vi "FPGA VI.vi"() -> ()   [LabVIEW 2015]
uses:
  Types/Injector.Timing.ctl
  Types/Injection.Core.Settings.ctl
  Types/Injection.Global.Settings.ctl
  <vilib>/rvi/eio/common/nirviEmuClasses.ctl
  <vilib>/Platform/TimedLoop/XDataNode/timing_clust.ctl
  <vilib>/Platform/TimedLoop/XDataNode/nitl_modes.ctl
  <vilib>/Platform/TimedLoop/XDataNode/wakeup.ctl
  Types/Injection.Core.Internal.Settings.ctl
  <vilib>/rvi/eio/common/nirviEmuTemplateMethod_errors.vi
  <vilib>/rvi/Emulation/niFpgaGetClockAttributes.vi
  <vilib>/rvi/Emulation/niFpgaSctlEmulationGetInTimedLoop.vi
  <vilib>/rvi/Emulation/niFpgaEmulationReportErrorSimple.vi
  <vilib>/rvi/Emulation/niFpgaCriticalErrorInLSC.vi
  <vilib>/rvi/DataTransferAndStorage/Container/Common/niFpgaContainerExecOnDevCompGetState.vi
  <vilib>/rvi/Emulation/niFpgaEmulationIsFPGAContextNoSignature.vi
  <vilib>/rvi/errors/niFpgaSetErrorForExecOnDevCompSimple.vi
  <vilib>/rvi/eio/common/nirviEmuReportErrorAndStop.vi
  <vilib>/rvi/DataTransferAndStorage/Container/Common/niFpgaContainerGetUniqueNameForEmu.vi
  <vilib>/rvi/FIFO/Fifo_Resource/nirvififoEmulationSetSize.vi
  <vilib>/rvi/FIFO/Fifo_Resource/nirviFifoEmulationQueueMgr.vi
  <instcachedir>/0/nirviFifoEmulationQueueMgr_E5CAEC123FF24DC58D834DCA3CDAA9B5.lvgen/nirviFifoEmulationQueueMgr_E5CAEC123FF24DC58D834DCA3CDAA9B5_010.vi
  <vilib>/rvi/FIFO/Fifo_Resource/nirvififoEmulationDetermineInputValidOut.vi
  <vilib>/rvi/FIFO/Fifo_Resource/nirvififoEmulationCreateLock.vi
  <vilib>/rvi/Emulation/niFpgaProcessEmulError.vi
  <vilib>/rvi/FIFO/Fifo_Resource/nirvififoEmulationObtainLock.vi
  <vilib>/rvi/FIFO/Fifo_Resource/nirvififoEmulationReleaseLock.vi
  <vilib>/rvi/occurrence/nirviWaitOnOccurrenceBase.vi
  <vilib>/rvi/errors/nirviReportUnexpectedCaseInternalError.vi
  <vilib>/rvi/errors/nirviReportUnexpectedCaseInternalError (U32).vi
  <vilib>/Utility/error.llb/Clear Errors.vi
  <vilib>/rvi/interface/RandomDataEmulation/niFpgaRandomDataHandleErrors.vi
  <instcachedir>/0/nirviFifoEmulationQueueMgr_E5CAEC123FF24DC58D834DCA3CDAA9B5.lvgen/nirviFifoEmulationQueueMgr_E5CAEC123FF24DC58D834DCA3CDAA9B5_008.vi
  <vilib>/eio/EIOGrowableMethodNode/genericMethod/EIOGrowableMethodNode.xnode
  <vilib>/rvi/eio/nirviEIOMethodImplementation/nirviEIOMethodImplementation.xnode
  <vilib>/rvi/eio/nirviErrorMerge/nirviErrorMerge.xnode
  <vilib>/eio/EIONode/EIONode.xnode
  <vilib>/Platform/TimedLoop/XDataNode/XDataNode.xnode
  <vilib>/rvi/DataTransferAndStorage/Container/XNode/niFpgaContainer.xnode
  <vilib>/rvi/FIFO/Fifo_Resource/niFpgaFifoEmulationRefIn.vi
  <vilib>/rvi/interface/RandomDataEmulation/nirviRandomDataFpgaReadWriteTemplate.vi
  <vilib>/Platform/TimedLoop/XDataNode/XDNodeRunTimeDep.lvlib
  <vilib>/rvi/eio/common/nirviEmuTemplateMethod_noerrors.vi
panel:
  out "Module Error":bool
  out "Sample Clock Ticks":u32
  out "Intermediate FIFO Write Timeout":bool
  in  "Settings.Global":T1={"Enable?"=FALSE, "Initial Voltage Threshold"=12.0, "Event Dwell Limit"=2000, "Voltage Gain"=1.0, "Current Gain"=1.0}
  in  "Settings.Index0.Injector0":T2
  in  "Settings.Index1.Injector1":T2
  in  "Settings.Index2.Injector2":T2
  in  "Settings.Index3.Injector3":T2
  in  "Settings.Index4.Injector4":T2
  in  "Settings.Index5.Injector5":T2
  in  "Settings.Timing":T3={"Injector Sample Period (Ticks)"=200}
  out "Acqusition Loop Ticks":u32
  in  "Settings.DMA":cluster{"# of Injectors":u8}={"# of Injectors"=6}
  out "Host DMA Out?":bool
  out "Intermediate Time Out?":bool
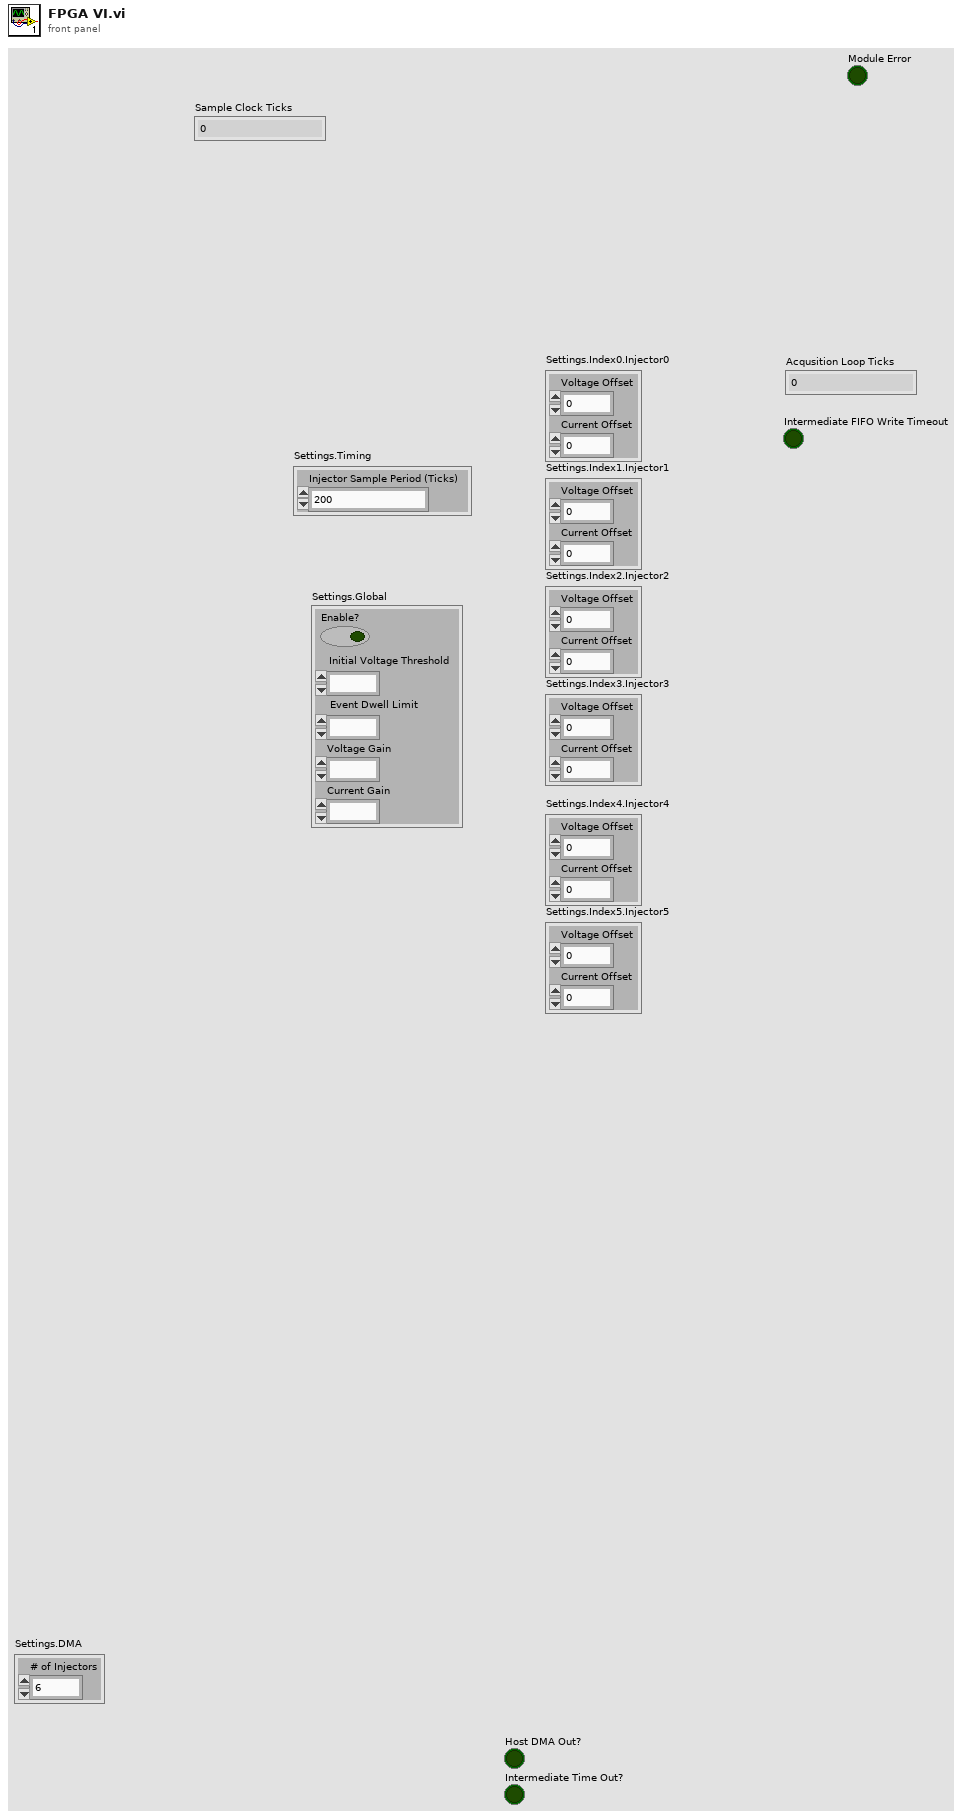
[diagram p1: front panel]
types:
  T1 = typedef "Injection.Global.Settings.ctl" = cluster{"Enable?":bool, "Initial Voltage Threshold":fxp<+/-,32,8>, "Event Dwell Limit":u16, "Voltage Gain":fxp<+/-,32,8>, "Current Gain":fxp<+/-,32,8>}
  T2 = typedef "Injection.Core.Settings.ctl" = cluster{"Voltage Offset":fxp<+/-,32,8>, "Current Offset":fxp<+/-,32,8>}
  T3 = typedef "Injector.Timing.ctl" = cluster{"Injector Sample Period (Ticks)":u32}
  T4 = typedef "nirviEmuClasses.ctl" = enum16{"IO Read", "IO Write", "Method", "Property Read", "Property Write"}
  T5 = cluster{"Data.Samples":u32, "Injection.Period":u32, "Injector.Index":u8, "Iteration":u32}
  T6 = enum8{"Wait on Transfer", "Transfer Injector Index", "Transfer # of Samples", "Transfer Injection Period", "Transfer Data Samples"}
  T7 = typedef "XDNodeRunTimeDep.lvlib/timing_clust.ctl" = cluster{"Expected End [f-1]":u64, "Actual End [f-1]":u64, "Finished Late? [f-1]":bool, "Expected End [i-1]":u64, "Actual End [i-1]":u64, "Finished Late? [i-1]":bool, "Expected Start [i]":u64, "Actual Start [i]":u64, "Expected Start [f]":u64, "Actual Start [f]":u64, "Source Name":string, "Structure Name":string, "Period":i64, "Deadline":i64, "Offset":i64, "Start":i64, "Priority":i32, "Timeout":i32, "Mode":T8, "Wakeup Reason":T9, "Error":errorcluster, "Source Type":string, "Secondary Source Type":string, "Global End Time":u64, "Global Start Time":u64, "Frame Duration":u64, "Iteration Duration":u64, "Assigned CPU":i32, "I/O Scan Engine Mode":u32}
  T8 = typedef "XDNodeRunTimeDep.lvlib/nitl_modes.ctl" = enum32{"No Change", "Process missed periods, maintain original phase", "Discard missed periods, maintain original phase", "Process missed periods, ignore original phase", "Discard missed periods, ignore original phase"}
  T9 = typedef "XDNodeRunTimeDep.lvlib/wakeup.ctl" = enum32{"Normal", "Aborted", "Asynchronous wakeup", "Timing source error", "Timed loop error", "Timeout"}
  T10 = typedef "Injection.Core.Internal.Settings.ctl" = cluster{"Data FIFO":refnum<k21>, "Trigger FIFO":refnum<k21>}
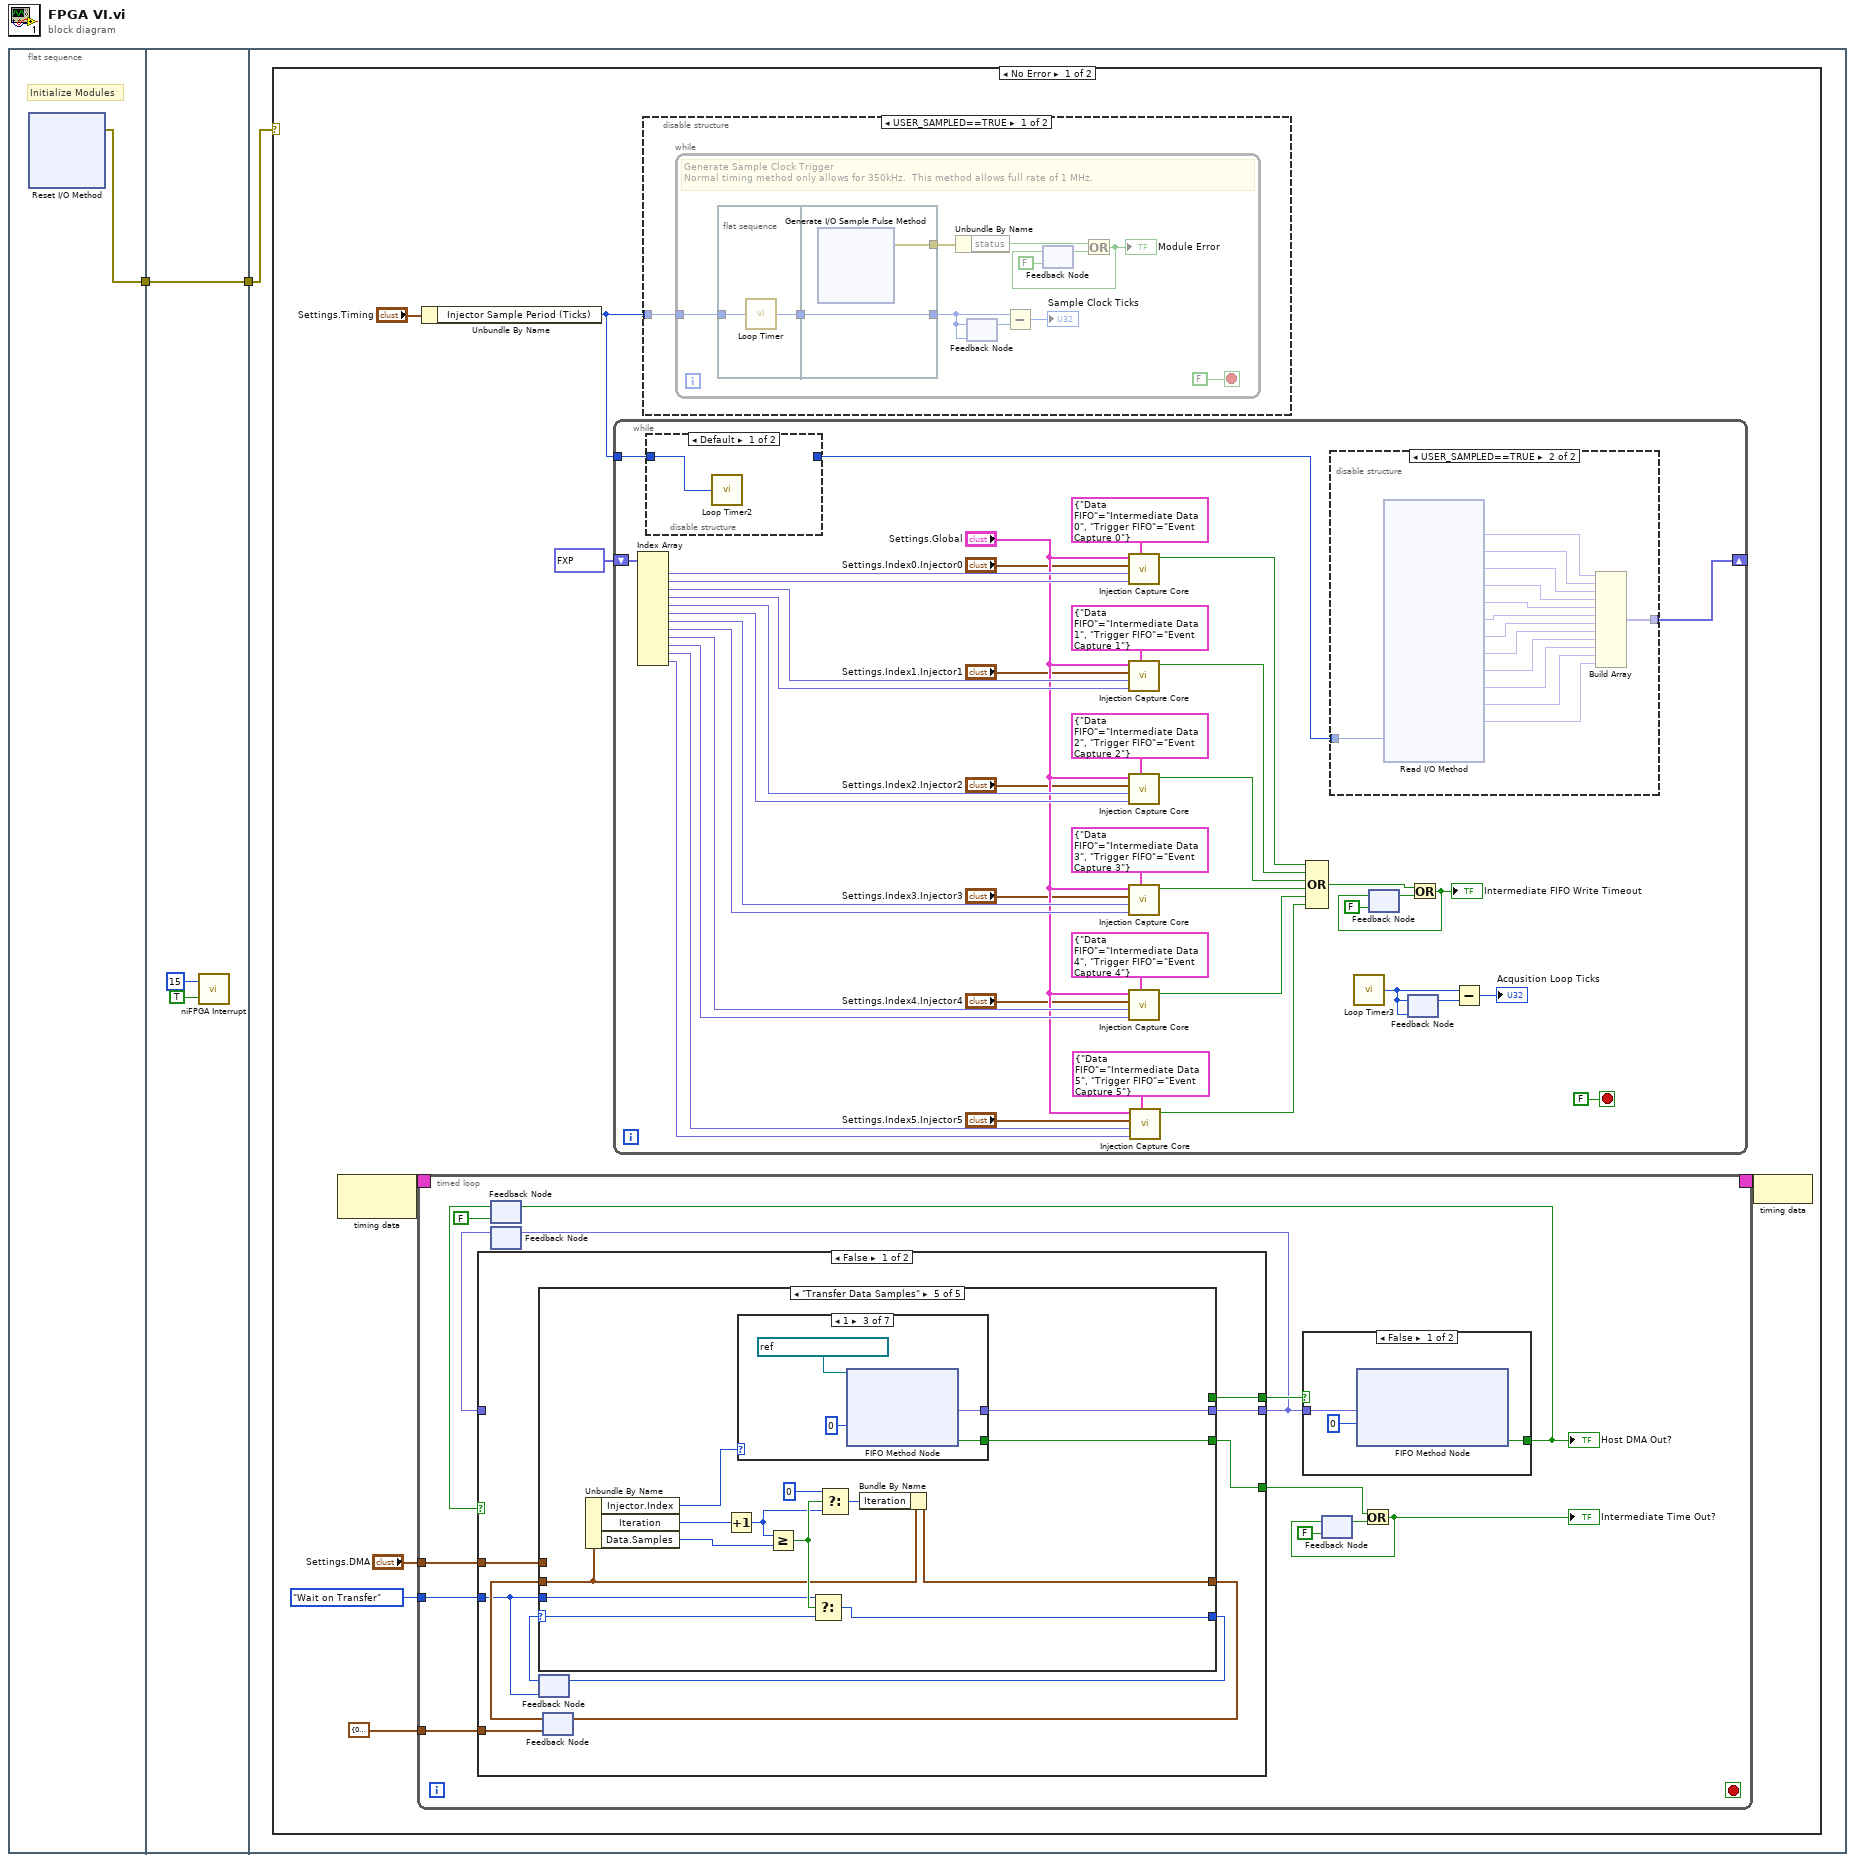
[diagram p0: block diagram]
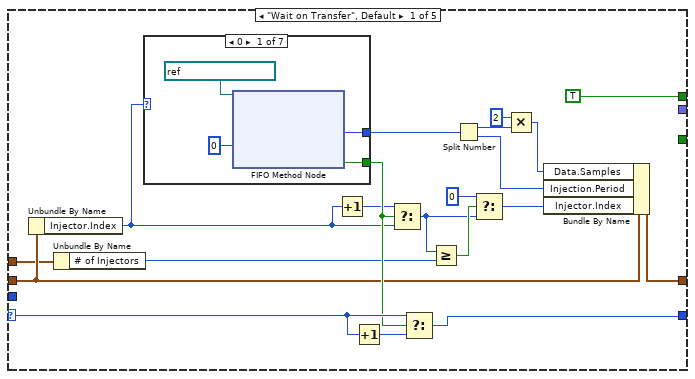
[diagram p2: hidden frame]
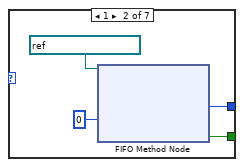
[diagram p3: hidden frame]
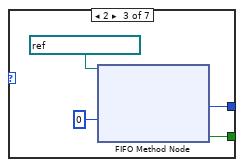
[diagram p4: hidden frame]
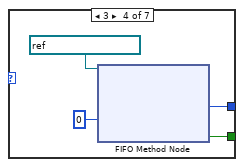
[diagram p5: hidden frame]
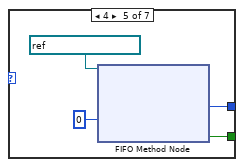
[diagram p6: hidden frame]
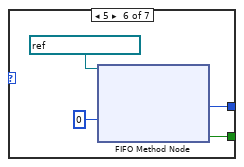
[diagram p7: hidden frame]
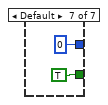
[diagram p8: hidden frame]
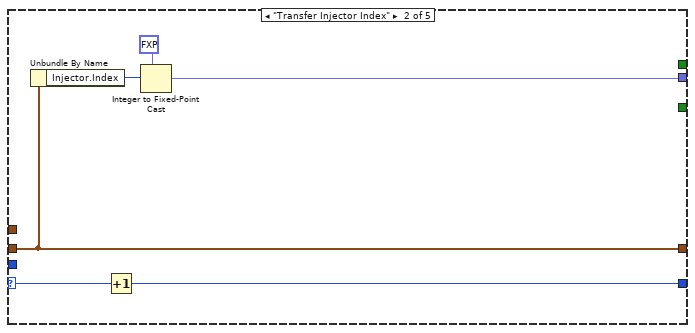
[diagram p9: hidden frame]
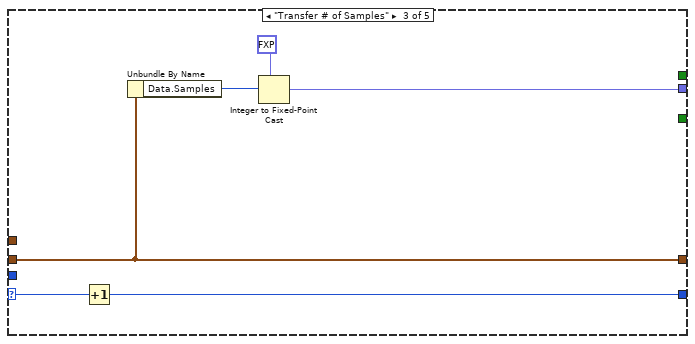
[diagram p10: hidden frame]
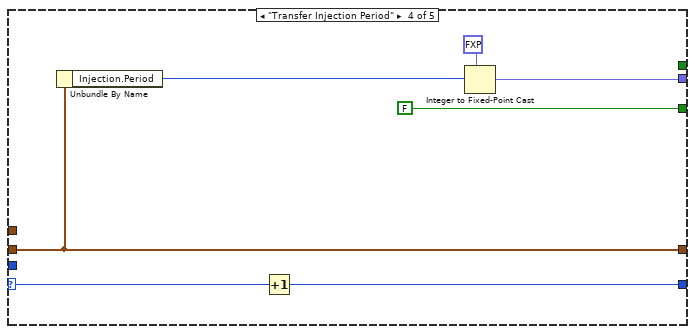
[diagram p11: hidden frame]
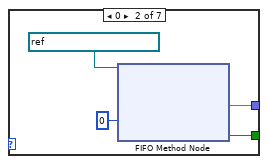
[diagram p13: hidden frame]
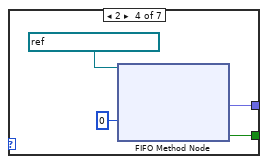
[diagram p14: hidden frame]
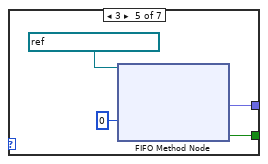
[diagram p15: hidden frame]
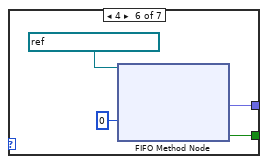
[diagram p16: hidden frame]
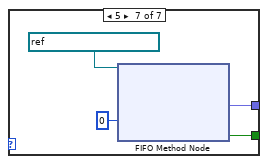
[diagram p17: hidden frame]
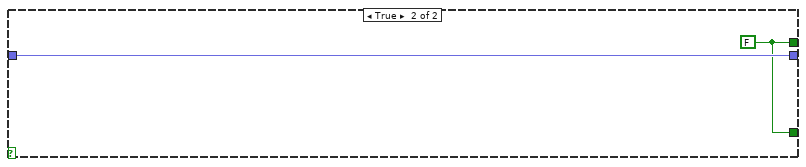
[diagram p18: hidden frame]
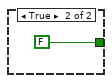
[diagram p19: hidden frame]
diagram:
  n1 = flat-sequence {
    tunnel: [w3] -> w2
    tunnel: w2 -> [w70]
    tunnel: [w70] -> w1
    tunnel: w1 -> [w71]
    frame #0 {
      # "Initialize Modules"
      n2 = xnode "Reset I/O Method"() -> ("error out"=w3:errorcluster)  [unwired: 4 in, 3 out]
    }
    frame #1 {
      n3 = call <vilib>:"niFPGA Interrupt.vi"("Wait Until Cleared (F)"=TRUE, "IRQ Number (0)"=u8 15) -> ()  [unwired: 1 in]
    }
    frame #2 {
      n4 = case shown="No Error" w71 {
        frame No Error {
          n5 = node-c288() -> (w79:T7)  [unwired: 1 in]
          n6 = timed-loop {
            timing: w79 -> [_]
            timing-out: [_] -> w78
            tunnel: "Settings.DMA" -> [w82]
            tunnel: T6."Wait on Transfer" -> [w81]
            tunnel: T5 {"Data.Samples"=0, "Injection.Period"=0, "Injector.Index"=0, "Iteration"=0} ("Local.Data") -> [w80]
            stop <- _ stop-if-true
            n7 = feedback #1(FALSE ("Timed Out?")) -> (w90:bool)
            n8 = feedback #2() -> (w87:fxp<+/-,32,8>)  [unwired: 1 in]
            n9 = case shown="False" w90 {
              tunnel: [w102 w207] -> w88
              tunnel: [w101 w206] -> w92
              tunnel: w81 -> [w94 _]
              tunnel: [w99 w206] -> w83
              tunnel: w82 -> [w98 _]
              tunnel: w80 -> [w95 _]
              tunnel: w87 -> [_ w207]
              frame False {
                n10 = feedback #3(w94) -> (w93:T6)
                n11 = feedback #4(w95) -> (w96:T5)
                n12 = case shown="\"Transfer Data Samples\"" w93 {
                  selector: w93 -> [w121 w154 w158 w166 w175]
                  tunnel: w96 -> [w112 w151 w156 w162 w173]
                  tunnel: [w120 w151 w156 w162 w172] -> w97
                  tunnel: [w119 w153 w157 w161 w174] -> w100
                  tunnel: [_ w150 w155 w165 w171] -> w102
                  tunnel: [TRUE _ _ _ _] -> w101
                  tunnel: w94 -> [_ _ _ _ w168]
                  tunnel: [_ _ _ FALSE ("Timed Out?") w170] -> w99
                  tunnel: w98 -> [w109 _ _ _ _]
                  frame "Wait on Transfer", Default {
                    n13 = Unbundle By Name(w112) -> ("Injector.Index"=w111:u8)
                    n14 = Unbundle By Name(w109) -> ("# of Injectors"=w108:u8)
                    n15 = case shown="0" w111 {
                      tunnel: [w125 w129 w133 w137 w141 w145 u64 0 ("Element")] -> w107
                      tunnel: [w124 w128 w132 w136 w140 w144 TRUE ("Timed Out?")] -> w117
                      frame 0 {
                        n16 = xnode ("FIFO Method Node")("Timeout"=0, "FIFO In"=refnum<k21> "Event Capture 0") -> ("Element"=w125:u64, "Timed Out?"=w124:bool)  [unwired: 1 out]
                      }
                      frame 1 {
                        n17 = xnode ("FIFO Method Node")("Timeout"=0, "FIFO In"=refnum<k21> "Event Capture 1") -> ("Element"=w129:u64, "Timed Out?"=w128:bool)  [unwired: 1 out]
                      }
                      frame 2 {
                        n18 = xnode ("FIFO Method Node")("Timeout"=0, "FIFO In"=refnum<k21> "Event Capture 2") -> ("Element"=w133:u64, "Timed Out?"=w132:bool)  [unwired: 1 out]
                      }
                      frame 3 {
                        n19 = xnode ("FIFO Method Node")("Timeout"=0, "FIFO In"=refnum<k21> "Event Capture 3") -> ("Element"=w137:u64, "Timed Out?"=w136:bool)  [unwired: 1 out]
                      }
                      frame 4 {
                        n20 = xnode ("FIFO Method Node")("Timeout"=0, "FIFO In"=refnum<k21> "Event Capture 4") -> ("Element"=w141:u64, "Timed Out?"=w140:bool)  [unwired: 1 out]
                      }
                      frame 5 {
                        n21 = xnode ("FIFO Method Node")("Timeout"=0, "FIFO In"=refnum<k21> "Event Capture 5") -> ("Element"=w145:u64, "Timed Out?"=w144:bool)  [unwired: 1 out]
                      }
                      frame Default {
                      }
                    }
                    n22 = Increment(x=w111) -> (x+1=w116:u8)
                    n23 = Increment(x=w121) -> (x+1=w122:T6)
                    n24 = Select(t=w116, s=w117, f=w111) -> (s? t:f=w114:u8)
                    n25 = Select(t=w121, s=w117, f=w122) -> (s? t:f=w119:T6)
                    n26 = Greater Or Equal?(x=w114, y=w108) -> (x >= y?=w115:bool)
                    n27 = Split Number(x=w107) -> (hi(x)=w106:u32, lo(x)=w105:u32)
                    n28 = Select(t=u8 0, s=w115, f=w114) -> (s? t:f=w110:u8)
                    n29 = Multiply(x=u32 2, y=w106) -> (x*y=w103:u32)
                    n30 = Bundle By Name(cluster=w112, "Data.Samples"=w103, "Injection.Period"=w105, "Injector.Index"=w110) -> (w120:T5)
                  }
                  frame "Transfer Injector Index" {
                    n31 = Unbundle By Name(w151) -> ("Injector.Index"=w152:u8)
                    n32 = Increment(x=w154) -> (x+1=w153:T6)
                    n33 = Integer to Fixed-Point Cast(fixed-point type=fxp<+/-,32,8> 0.0, integer=w152) -> (fixed-point=w150:fxp<+/-,32,8>)
                  }
                  frame "Transfer # of Samples" {
                    n34 = Increment(x=w158) -> (x+1=w157:T6)
                    n35 = Unbundle By Name(w156) -> ("Data.Samples"=w159:u32)
                    n36 = Integer to Fixed-Point Cast(fixed-point type=fxp<+/-,32,8> 0.0, integer=w159) -> (fixed-point=w155:fxp<+/-,32,8>)
                  }
                  frame "Transfer Injection Period" {
                    n37 = Unbundle By Name(w162) -> ("Injection.Period"=w164:u32)
                    n38 = Increment(x=w166) -> (x+1=w161:T6)
                    n39 = Integer to Fixed-Point Cast(fixed-point type=fxp<+/-,32,8> 0.0, integer=w164) -> (fixed-point=w165:fxp<+/-,32,8>)
                  }
                  frame "Transfer Data Samples" {
                    n40 = Unbundle By Name(w173) -> ("Injector.Index"=w181:u8, "Iteration"=w176:u32, "Data.Samples"=w169:u32)
                    n41 = Increment(x=w176) -> (x+1=w178:u32)
                    n42 = case shown="1" w181 {
                      tunnel: [_ w184 w188 w192 w196 w200 w204] -> w171
                      tunnel: [_ w183 w187 w191 w195 w199 w203] -> w170
                      frame Default {
                      }
                      frame 0 {
                        n43 = xnode ("FIFO Method Node")("Timeout"=0, "FIFO In"=refnum<k21> "Intermediate Data 0" ("Voltage FIFO")) -> ("Element"=w184:fxp<+/-,32,8>, "Timed Out?"=w183:bool)  [unwired: 1 out]
                      }
                      frame 1 {
                        n44 = xnode ("FIFO Method Node")("Timeout"=0, "FIFO In"=refnum<k21> "Intermediate Data 1" ("Voltage FIFO")) -> ("Element"=w188:fxp<+/-,32,8>, "Timed Out?"=w187:bool)  [unwired: 1 out]
                      }
                      frame 2 {
                        n45 = xnode ("FIFO Method Node")("Timeout"=0, "FIFO In"=refnum<k21> "Intermediate Data 2" ("Voltage FIFO")) -> ("Element"=w192:fxp<+/-,32,8>, "Timed Out?"=w191:bool)  [unwired: 1 out]
                      }
                      frame 3 {
                        n46 = xnode ("FIFO Method Node")("Timeout"=0, "FIFO In"=refnum<k21> "Intermediate Data 3" ("Voltage FIFO")) -> ("Element"=w196:fxp<+/-,32,8>, "Timed Out?"=w195:bool)  [unwired: 1 out]
                      }
                      frame 4 {
                        n47 = xnode ("FIFO Method Node")("Timeout"=0, "FIFO In"=refnum<k21> "Intermediate Data 4" ("Voltage FIFO")) -> ("Element"=w200:fxp<+/-,32,8>, "Timed Out?"=w199:bool)  [unwired: 1 out]
                      }
                      frame 5 {
                        n48 = xnode ("FIFO Method Node")("Timeout"=0, "FIFO In"=refnum<k21> "Intermediate Data 5" ("Voltage FIFO")) -> ("Element"=w204:fxp<+/-,32,8>, "Timed Out?"=w203:bool)  [unwired: 1 out]
                      }
                    }
                    n49 = Greater Or Equal?(x=w178, y=w169) -> (x >= y?=w180:bool)
                    n50 = Select(t=w168, s=w180, f=w175) -> (s? t:f=w174:T6)
                    n51 = Select(t=u32 0, s=w180, f=w178) -> (s? t:f=w177:u32)
                    n52 = Bundle By Name(cluster=w173, "Iteration"=w177) -> (w172:T5)
                  }
                }
                n53 = feedback-in #3(w100) -> ()
                n54 = feedback-in #4(w97) -> ()
              }
              frame True {
                w206 = FALSE
              }
            }
            n55 = feedback-in #2(w88) -> ()
            n56 = case shown="False" w92 {
              tunnel: w88 -> [w209 _]
              tunnel: [w208 FALSE ("Timed Out?")] -> w91
              frame False {
                n57 = xnode ("FIFO Method Node")("Element"=w209, "Timeout"=0) -> ("Timed Out?"=w208:bool)  [unwired: 1 in, 1 out]
              }
              frame True {
              }
            }
            "Host DMA Out?" <- w91
            n58 = feedback-in #1(w91) -> ()
            n59 = feedback #5(FALSE ("Timed Out?")) -> (w85:bool)
            n60 = Or(x=w83, y=w85) -> (x .or. y?=w84:bool)
            "Intermediate Time Out?" <- w84
            n61 = feedback-in #5(w84) -> ()
          }
          n62 = Unbundle By Name("Settings.Timing") -> ("Injector Sample Period (Ticks)"=w72:u32)
          n63 = while {
            shift-right: [w303] -> _
            shift-left: fxp<+/-,24,5>[] [0.0, 0.0, 0.0, 0.0, 0.0, 0.0, 0.0, 0.0, 0.0, 0.0, 0.0, 0.0] -> [w319]
            tunnel: w72 -> [w302]
            stop <- FALSE stop-if-true
            n64 = Index Array(array=w319) -> (element #1=w330:fxp<+/-,24,5>, element #2=w331:fxp<+/-,24,5>, element #3=w328:fxp<+/-,24,5>, element #4=w329:fxp<+/-,24,5>, element #5=w326:fxp<+/-,24,5>, element #6=w327:fxp<+/-,24,5>, element #7=w324:fxp<+/-,24,5>, element #8=w325:fxp<+/-,24,5>, element #9=w322:fxp<+/-,24,5>, element #10=w323:fxp<+/-,24,5>, element #11=w320:fxp<+/-,24,5>, element #12=w321:fxp<+/-,24,5>)  [unwired: 12 in]
            n65 = disable-structure shown="Default" {
              disable-tunnel: w302 -> [w339 w340]
              disable-tunnel: [_ w340] -> w301
              frame condition #0 (active) {
                n66 = call "Loop Timer2"("Count(Ticks)"=w339) -> ()  [unwired: 1 out]
              }
              frame condition #1 {
              }
            }
            n67 = call "Injection Capture Core.vi"("FIFOs"=T10 {"Data FIFO"="Intermediate Data 0", "Trigger FIFO"="Event Capture 0"} ("InjectorCore.Settings"), "Current (PreScaled)"=w331, "Voltage (PreScaled)"=w330, "Settings.Index<#>.<UserName>"="Settings.Index0.Injector0", "Settings.Global"="Settings.Global") -> ("Intermediate FIFO Timeout?"=w338:bool)  [unwired: 4 in, 2 out]
            n68 = call "Injection Capture Core.vi"("FIFOs"=T10 {"Data FIFO"="Intermediate Data 1", "Trigger FIFO"="Event Capture 1"} ("InjectorCore.Settings"), "Current (PreScaled)"=w329, "Voltage (PreScaled)"=w328, "Settings.Index<#>.<UserName>"="Settings.Index1.Injector1", "Settings.Global"="Settings.Global") -> ("Intermediate FIFO Timeout?"=w337:bool)  [unwired: 4 in, 2 out]
            n69 = call "Injection Capture Core.vi"("FIFOs"=T10 {"Data FIFO"="Intermediate Data 2", "Trigger FIFO"="Event Capture 2"} ("InjectorCore.Settings"), "Current (PreScaled)"=w327, "Voltage (PreScaled)"=w326, "Settings.Index<#>.<UserName>"="Settings.Index2.Injector2", "Settings.Global"="Settings.Global") -> ("Intermediate FIFO Timeout?"=w336:bool)  [unwired: 4 in, 2 out]
            n70 = call "Injection Capture Core.vi"("FIFOs"=T10 {"Data FIFO"="Intermediate Data 3", "Trigger FIFO"="Event Capture 3"} ("InjectorCore.Settings"), "Current (PreScaled)"=w325, "Voltage (PreScaled)"=w324, "Settings.Index<#>.<UserName>"="Settings.Index3.Injector3", "Settings.Global"="Settings.Global") -> ("Intermediate FIFO Timeout?"=w335:bool)  [unwired: 4 in, 2 out]
            n71 = call "Injection Capture Core.vi"("FIFOs"=T10 {"Data FIFO"="Intermediate Data 4", "Trigger FIFO"="Event Capture 4"} ("InjectorCore.Settings"), "Current (PreScaled)"=w323, "Voltage (PreScaled)"=w322, "Settings.Index<#>.<UserName>"="Settings.Index4.Injector4", "Settings.Global"="Settings.Global") -> ("Intermediate FIFO Timeout?"=w334:bool)  [unwired: 4 in, 2 out]
            n72 = call "Injection Capture Core.vi"("FIFOs"=T10 {"Data FIFO"="Intermediate Data 5", "Trigger FIFO"="Event Capture 5"} ("InjectorCore.Settings"), "Current (PreScaled)"=w321, "Voltage (PreScaled)"=w320, "Settings.Index<#>.<UserName>"="Settings.Index5.Injector5", "Settings.Global"="Settings.Global") -> ("Intermediate FIFO Timeout?"=w333:bool)  [unwired: 4 in, 2 out]
            n73 = Compound Arithmetic op=OR(w338, w337, w336, w335, w334, w333) -> (w308:bool)
            n74 = disable-structure shown="USER_SAMPLED==TRUE" {
              disable-tunnel: [w352 w366] -> w303
              disable-tunnel: w301 -> [_ w354]
              frame condition #0 (active) {
                n75 = xnode "FPGA I/O Node"() -> ("Mod1/AI0"=w353:fxp<+/-,24,5>, "Mod1/AI1"=w351:fxp<+/-,24,5>, "Mod1/AI2"=w350:fxp<+/-,24,5>, "Mod1/AI3"=w349:fxp<+/-,24,5>, "Mod2/AI0"=w348:fxp<+/-,24,5>, "Mod2/AI1"=w347:fxp<+/-,24,5>, "Mod2/AI2"=w346:fxp<+/-,24,5>, "Mod2/AI3"=w345:fxp<+/-,24,5>, "Mod3/AI0"=w344:fxp<+/-,24,5>, "Mod3/AI1"=w343:fxp<+/-,24,5>, "Mod3/AI2"=w342:fxp<+/-,24,5>, "Mod3/AI3"=w341:fxp<+/-,24,5>)  [unwired: 12 in, 12 out]
                n76 = Build Array(w353, w351, w350, w349, w348, w347, w346, w345, w344, w343, w342, w341) -> (w352:fxp<+/-,24,5>[])
              }
              frame condition #1 {
                n77 = xnode "Read I/O Method"("Timeout"=w354) -> ("Mod1/AI0"=w367:fxp<+/-,24,5>, "Mod1/AI1"=w365:fxp<+/-,24,5>, "Mod1/AI2"=w364:fxp<+/-,24,5>, "Mod1/AI3"=w363:fxp<+/-,24,5>, "Mod2/AI0"=w362:fxp<+/-,24,5>, "Mod2/AI1"=w361:fxp<+/-,24,5>, "Mod2/AI2"=w360:fxp<+/-,24,5>, "Mod2/AI3"=w359:fxp<+/-,24,5>, "Mod3/AI0"=w358:fxp<+/-,24,5>, "Mod3/AI1"=w357:fxp<+/-,24,5>, "Mod3/AI2"=w356:fxp<+/-,24,5>, "Mod3/AI3"=w355:fxp<+/-,24,5>)  [unwired: 13 in, 14 out]
                n78 = Build Array(w367, w365, w364, w363, w362, w361, w360, w359, w358, w357, w356, w355) -> (w366:fxp<+/-,24,5>[])
              }
            }
            n79 = call "Loop Timer3"() -> ("Tick Count(Ticks)"=w304:u32)  [unwired: 1 in]
            n80 = feedback #6(FALSE ("Timed Out?")) -> (w309:bool)
            n81 = feedback-in #7(w304) -> ()
            n82 = feedback #7(w304) -> (w306:u32)
            n83 = Or(x=w308, y=w309) -> (x .or. y?=w307:bool)
            "Intermediate FIFO Write Timeout" <- w307
            n84 = feedback-in #6(w307) -> ()
            n85 = Subtract(x=w304, y=w306) -> (x-y=→"Acqusition Loop Ticks":u32)
          }
          n86 = disable-structure shown="USER_SAMPLED==TRUE" {
            disable-tunnel: w72 -> [w216 _]
            frame condition #0 {
              n87 = while {
                tunnel: w216 -> [w226]
                stop <- FALSE stop-if-true
                # "Generate Sample Clock Trigger\nNormal timing method only allows for 350kHz.  This method allows full rate of 1 MHz."
                n88 = flat-sequence {
                  tunnel: w226 -> [w229]
                  tunnel: [w228] -> w217
                  tunnel: [w231] -> w227
                  tunnel: [w230] -> w218
                  tunnel: w217 -> [w230]
                  frame #0 {
                    n89 = call "Loop Timer"("Count(Ticks)"=w229) -> ("Tick Count(Ticks)"=w228:u32)
                  }
                  frame #1 {
                    n90 = xnode "Generate I/O Sample Pulse Method"() -> ("error out"=w231:errorcluster)  [unwired: 4 in, 3 out]
                  }
                }
                n91 = Unbundle By Name(w227) -> ("status"=w219:bool)
                n92 = feedback #8(w218) -> (w224:u32)
                n93 = feedback-in #8(w218) -> ()
                n94 = Subtract(x=w218, y=w224) -> (x-y=→"Sample Clock Ticks":u32)
                n95 = feedback #9(FALSE ("Timed Out?")) -> (w221:bool)
                n96 = Or(x=w219, y=w221) -> (x .or. y?=w220:bool)
                "Module Error" <- w220
                n97 = feedback-in #9(w220) -> ()
              }
            }
            frame condition #1 (active) {
            }
          }
          n98 = node-c288(w78) -> ()
        }
        frame Error {
        }
      }
    }
  }
